vi "FT10_Semi-Auto Parse Commands.vi"(11 "Semi-Auto Cluster":T4) -> (3 "appended array":T3[](array[typedef]))   [LabVIEW 2024]
doc: "Turn cluster commands into message array that can be sent to Message Handling Loop queue.\n\nMessage order: Set config, Set mode, Set power level, Activate port, Read & Wait, Deactivate port"
uses:
  Controls/Control_Semi-Auto Cluster.ctl
  Controls/Control_Semi-Auto Unitherm Load.ctl
  Controls/Control_Semi-Auto Port.ctl
  Controls/Control_Semi-Auto Mode.ctl
  Controls/Control_Semi-Auto Power Level.ctl
  Controls/Control_Semi-Auto Activation Duration.ctl
  Controls/Control_Command Cluster.ctl
panel:
  out "Mode":T1
  out "Port":T2
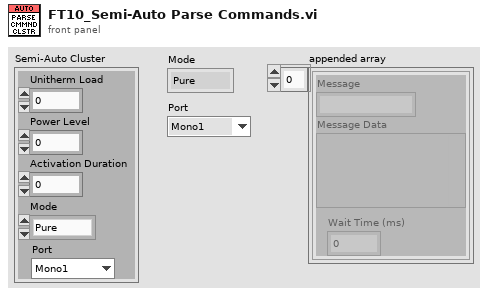
[diagram p1: front panel]
types:
  T1 = typedef "Control_Semi-Auto Mode.ctl" = enum16{"Pure", "Blend", "Spray", "Fulgerate", "Standard", "Macro", "Precision", "Ligasure", "Error"}
  T2 = typedef "Control_Semi-Auto Port.ctl" = enum16{"Mono1", "Mono2", "Bipolar", "Ligasure", "Error"}
  T3 = typedef "Control_Command Cluster.ctl" = cluster{"Message":string, "Message Data":variant, "Wait Time (ms)":i32}
  T4 = typedef "Control_Semi-Auto Cluster.ctl" = cluster{"Unitherm Load":T5, "Port":T2, "Mode":T1, "Power Level":T6, "Activation Duration":T7}
  T5 = typedef "Control_Semi-Auto Unitherm Load.ctl" = i32
  T6 = typedef "Control_Semi-Auto Power Level.ctl" = dbl
  T7 = typedef "Control_Semi-Auto Activation Duration.ctl" = i32
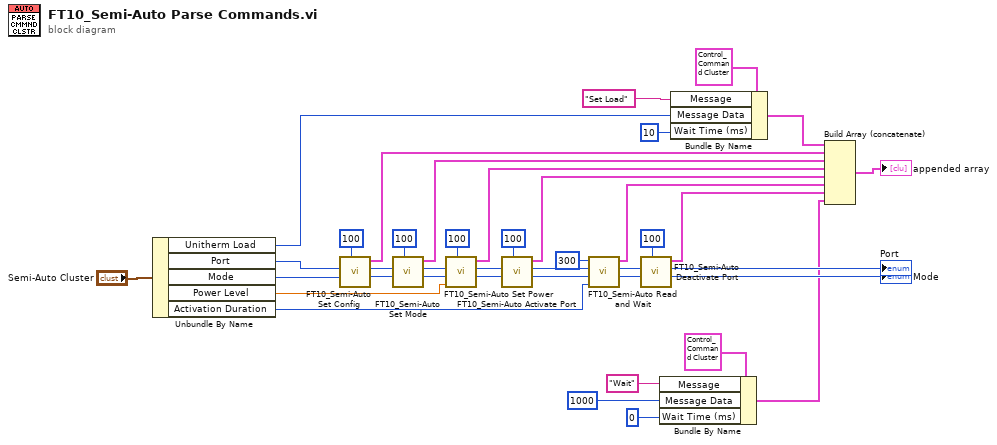
[diagram p0: block diagram]
diagram:
  n1 = Unbundle By Name("Semi-Auto Cluster") -> ("Unitherm Load"=w36:T5, "Port"=w33:T2, "Mode"=w32:T1, "Power Level"=w15:T6, "Activation Duration"=w16:T7)
  n2 = call "FT10_Semi-Auto Set Config.vi"("Wait Time (ms)"=100, "Mode in"=w32, "Port in"=w33) -> ("Mode out"=w30:T1, "Port out"=w31:T2, "output cluster"=w29:T3)  [unwired: 6 in]
  n3 = call "FT10_Semi-Auto Set Mode.vi"("Wait Time (ms)"=100, "Mode in"=w30, "Port in"=w31) -> ("Mode out"=w13:T1, "Port out"=w14:T2, "Command Cluster"=w28:T3)  [unwired: 6 in]
  n4 = call "FT10_Semi-Auto Set Power.vi"("Wait Time (ms)"=100, "Power Level"=w15, "Mode in"=w13, "Port in"=w14) -> ("Mode out"=w11:T1, "Port out"=w12:T2, "output cluster"=w7:T3)  [unwired: 5 in]
  n5 = call "FT10_Semi-Auto Activate Port.vi"("Wait Time (ms)"=100, "Mode in"=w11, "Port in"=w12) -> ("Mode out"=w22:T1, "Port out"=w21:T2, "Command Cluster"=w8:T3)  [unwired: 6 in]
  n6 = call "FT10_Semi-Auto Read and Wait.vi"("Activation Duration"=w16, "Mode in"=w22, "Port in"=w21, "Read Frequency"=300) -> ("Mode out"=w18:T1, "Port out"=w19:T2, "Command Cluster Array"=w9:T3[])  [unwired: 5 in]
  n7 = call "FT10_Semi-Auto Deactivate Port.vi"("Wait Time (ms)"=100, "Mode in"=w18, "Port in"=w19) -> ("Mode out"=→"Mode":T1, "Port out"=→"Port":T2, "Command Cluster"=w10:T3)  [unwired: 6 in]
  n8 = Bundle By Name(cluster=T3 {"Message"="", "Message Data"=variant, "Wait Time (ms)"=0}, "Message"="Wait", "Message Data"=1000 ("Wait Time (ms)"), "Wait Time (ms)"=0) -> (w1:T3)
  n9 = Bundle By Name(cluster=T3 {"Message"="", "Message Data"=variant, "Wait Time (ms)"=0}, "Message"="Set Load", "Message Data"=w36, "Wait Time (ms)"=10) -> (w39:T3)
  n10 = Build Array (concatenate)(w39, w29, w28, w7, w8, w9, w10, w1) -> (→"appended array":T3[])
